vi "Read alarm XML.vi"(0 "map in":T2) -> (7 "map out":T1, 8 "data":T3, 9 "change?":bool)   [LabVIEW 2016, in "Alarm interface.lvlib"]
uses:
  Alarm interface.lvlib
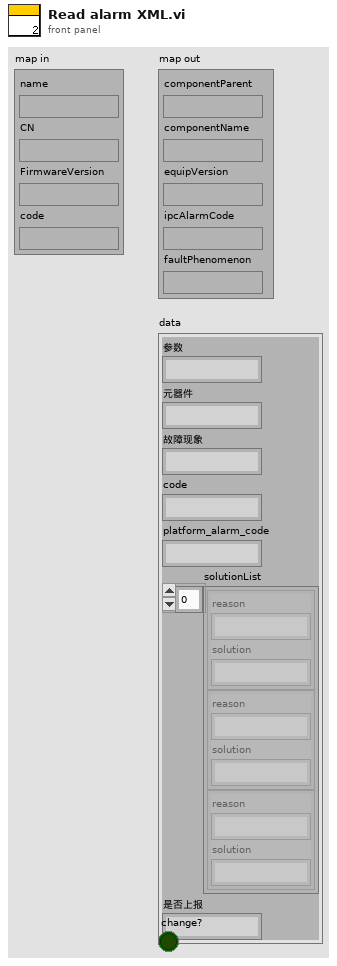
[diagram p1: front panel]
types:
  T1 = typedef "Alarm interface.lvlib/map out.ctl" = cluster{"componentParent":string, "componentName":string, "equipVersion":string, "ipcAlarmCode":string, "faultPhenomenon":string}
  T2 = typedef "Alarm interface.lvlib/map in.ctl" = cluster{"name":string, "CN":string, "FirmwareVersion":string, "code":string}
  T3 = typedef "Alarm interface.lvlib/报警短信语音交互.ctl" = cluster{"参数":string, "元器件":string, "故障现象":string, "code":string, "platform_alarm_code":string, "solutionList":cluster{"reason":string, "solution":string}[], "是否上报":string}
  T4 = cluster{"componentParentPath":string, "componentParentName":string, "componentName":string, "faultName":string, "equipVersion":string, "alarmCode":string, "ipcAlarmCode":string, "solutionList":cluster{"id":string, "faultId":string, "reason":string, "dataPhenomenon":string, "analysis":string, "solution":string}[]}
  T5 = cluster{"id":string, "faultId":string, "reason":string, "dataPhenomenon":string, "analysis":string, "solution":string}[]
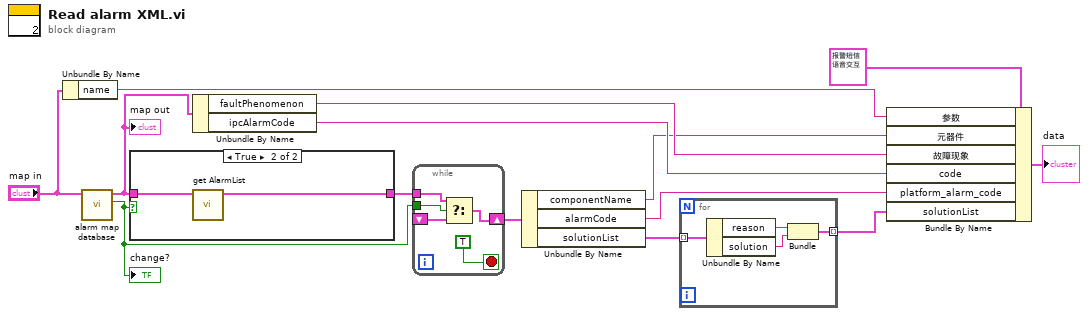
[diagram p0: block diagram]
diagram:
  n1 = Unbundle By Name("map in") -> ("name"=w5:string)
  n2 = call "alarm map database.vi"("map in"="map in") -> ("change?"=w7:bool, "map out"=w1:T1)  [unwired: 8 in, 1 out]
  "map out" <- w1
  "change?" <- w7
  n3 = case shown="True" w7 {
    tunnel: [_ w16] -> w13
    tunnel: w1 -> [_ w15]
    frame False {
    }
    frame True {
      n4 = call "get AlarmList.vi"("map out"=w15) -> ("alarm"=w16:T4)  [unwired: 9 in, 1 out]
    }
  }
  n5 = Unbundle By Name(w1) -> ("faultPhenomenon"=w3:string, "ipcAlarmCode"=w4:string)
  n6 = while {
    tunnel: w13 -> [w20]
    shift-right: [w18] -> w12
    shift-left: _ -> [w19]
    tunnel: w7 -> [w21]
    stop <- TRUE stop-if-true
    n7 = Select(t=w20, s=w21, f=w19) -> (s? t:f=w18:T4)
  }
  n8 = Unbundle By Name(w12) -> ("componentName"=w2:string, "alarmCode"=w11:string, "solutionList"=w10:T5)
  n9 = for {
    tunnel: w10 -> [w25] mode=indexing
    tunnel: [w22] -> w8 mode=indexing
    n10 = Unbundle By Name(w25) -> ("reason"=w24:string, "solution"=w23:string)
    n11 = Bundle("reason"=w24, "solution"=w23) -> (w22:cluster{"reason":string, "solution":string})  [unwired: 1 in]
  }
  n12 = Bundle By Name(cluster=T3 {"参数"="", "元器件"="", "故障现象"="", "code"="", "platform_alarm_code"="", "solutionList"=[{"reason"="1、缺标液，", "solution"="1、检查标液口（标液是否用完，及附属管路气密性等），检查管路气密性"}, {"reason"="2、液位传感器异常", "solution"="2、更换液位传感器"}, {"reason"="3、蠕动泵故障或泵管老化导致无法正常抽液", "solution"="3、更换蠕动泵管或更换蠕动泵"}], "是否上报"=""} ("data"), "参数"=w5, "元器件"=w2, "故障现象"=w3, "code"=w4, "platform_alarm_code"=w11, "solutionList"=w8) -> (→"data":T3)
